vi "Robot Drive Teleop.vi"(9 "Drive Mode":enum16{"Tank Drive", "Arcade Drive"}(ring), 10 "RobotDriveDevRef":T1, 11 "Controller Mode":enum16{"X-Box Controller", "Joysticks"}(ring)) -> (2 "Publish Motors":bool, 3 "Motor Values":dbl[](array[numeric]))   [LabVIEW 2015]
uses:
  <vilib>/Rock Robotics/WPI/RobotDrive/WPI_RobotDriveDevRef.ctl
  <vilib>/Rock Robotics/WPI/MotorControl/WPI_MotorControlDeviceRef.ctl
  <vilib>/Rock Robotics/WPI/MotorControl/WPI_MotorControlType.ctl
  <vilib>/Rock Robotics/SystemInterfaces/DIO/FPGA_DIOPWMChannel.ctl
  <vilib>/Rock Robotics/WPI/PWM/WPI_PWMDeadband.ctl
  <vilib>/Rock Robotics/WPI/CAN/Jaguar/SubVIs/WPI_CANJaguar_ControlMode.ctl
  <vilib>/Rock Robotics/WPI/CAN/TalonSRX/WPI_CANTalonSRX_APIControlMode.ctl
  <vilib>/Rock Robotics/WPI/DriverStation/WPI_DriverStationDerivedRobotMode.ctl
  Robot Global Data.vi
  <vilib>/Rock Robotics/WPI/Utilities/WPI_GetSetVariantRefNum.vi
  <vilib>/Rock Robotics/Network Tables/NT Write Numeric Array.vi
  <vilib>/Rock Robotics/Network Tables/NT Write Boolean Array.vi
panel:
  in  "Buttons":bool[](array[boolean])
  in  "Axes":dbl[](array[numeric])
  in  "POVs":i16[](array[numeric])
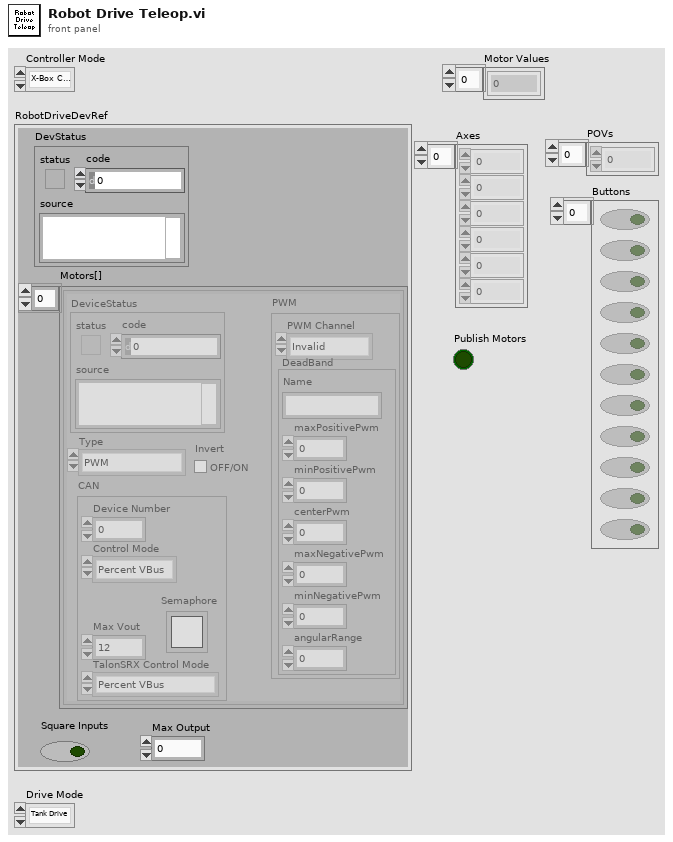
[diagram p1: front panel]
types:
  T1 = typedef "WPI_RobotDriveDevRef.ctl" = cluster{"DevStatus":errorcluster, "Motors[]":T2[], "Square Inputs":bool, "Max Output":dbl}
  T2 = typedef "WPI_MotorControlDeviceRef.ctl" = cluster{"DeviceStatus":errorcluster, "Type":T3, "PWM":cluster{"PWM Channel":T4, "DeadBand":T5}, "CAN":cluster{"Device Number":u8, "Control Mode":T6, "Semaphore":T7, "Max Vout":dbl, "TalonSRX Control Mode":T8}, "Invert":bool}
  T3 = typedef "WPI_MotorControlType.ctl" = enum16{"PWM", "CAN", "CANTalonSRX"}
  T4 = typedef "FPGA_DIOPWMChannel.ctl" = enum8{"PWM 0", "PWM 1", "PWM 2", "PWM 3", "PWM 4", "PWM 5", "PWM 6", "PWM 7", "PWM 8", "PWM 9", "PWM MXP 0", "PWM MXP 1", "PWM MXP 2", "PWM MXP 3", "PWM MXP 4", "PWM MXP 5", "PWM MXP 6", "PWM MXP 7", "PWM MXP 8", "PWM MXP 9", "Invalid"}
  T5 = typedef "WPI_PWMDeadband.ctl" = cluster{"Name":string, "maxPositivePwm":i32, "minPositivePwm":i32, "centerPwm":i32, "maxNegativePwm":i32, "minNegativePwm":i32, "angularRange":u16}
  T6 = typedef "WPI_CANJaguar_ControlMode.ctl" = enum8{"Percent VBus", "Current", "Speed", "Position", "Voltage"}
  T7 = typedef "Semaphore RefNum" = refnum<k1>
  T8 = typedef "WPI_CANTalonSRX_APIControlMode.ctl" = enum8{"Percent VBus", "Speed", "Position", "Slave", "Unchanged / Invalid", "Voltage Compensation", "Current", "Motion Profile"}
  T9 = cluster{"Drive Operation":enum16{"Turn Robot", "Drive Straight for Time"}, "Turn Angle":dbl, "Drive Time":dbl, "Forward Speed":dbl}
  T10 = typedef "WPI_DriverStationDerivedRobotMode.ctl" = enum16{"Init", "Execute", "Stop"}
  T11 = typedef "WPI_JoystickDevRef.ctl" = cluster{"Device":T12}
  T12 = typedef "WPI_JoystickDeviceEnum.ctl" = enum16{"USB 0", "USB 1", "USB 2", "USB 3", "USB 4", "USB 5"}
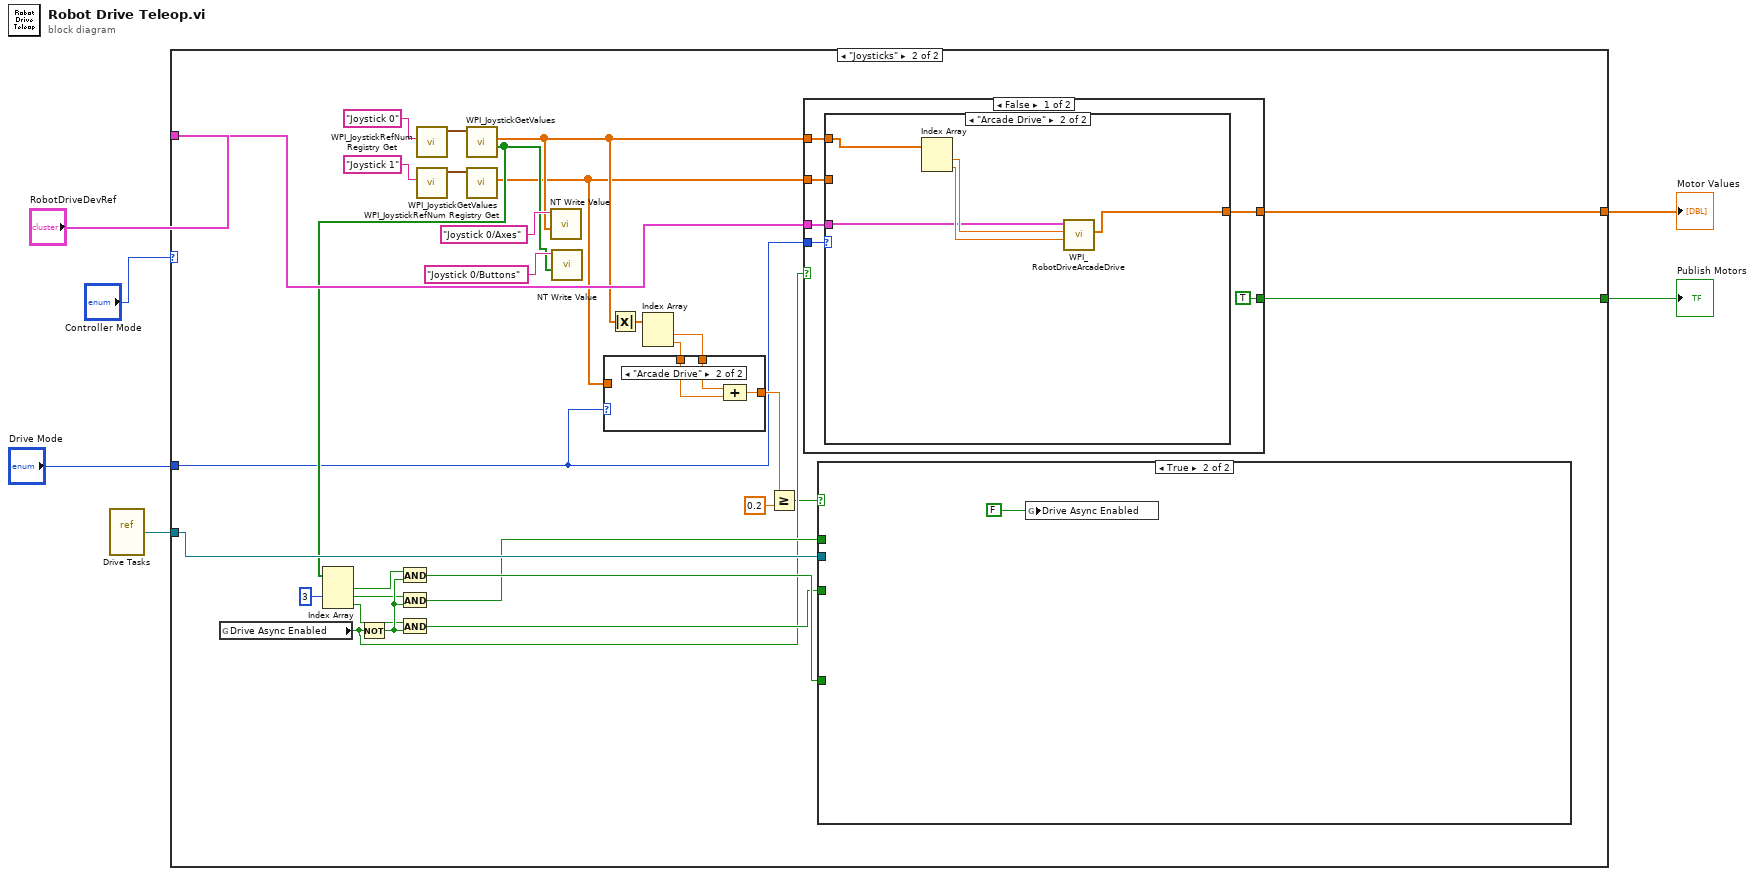
[diagram p0: block diagram]
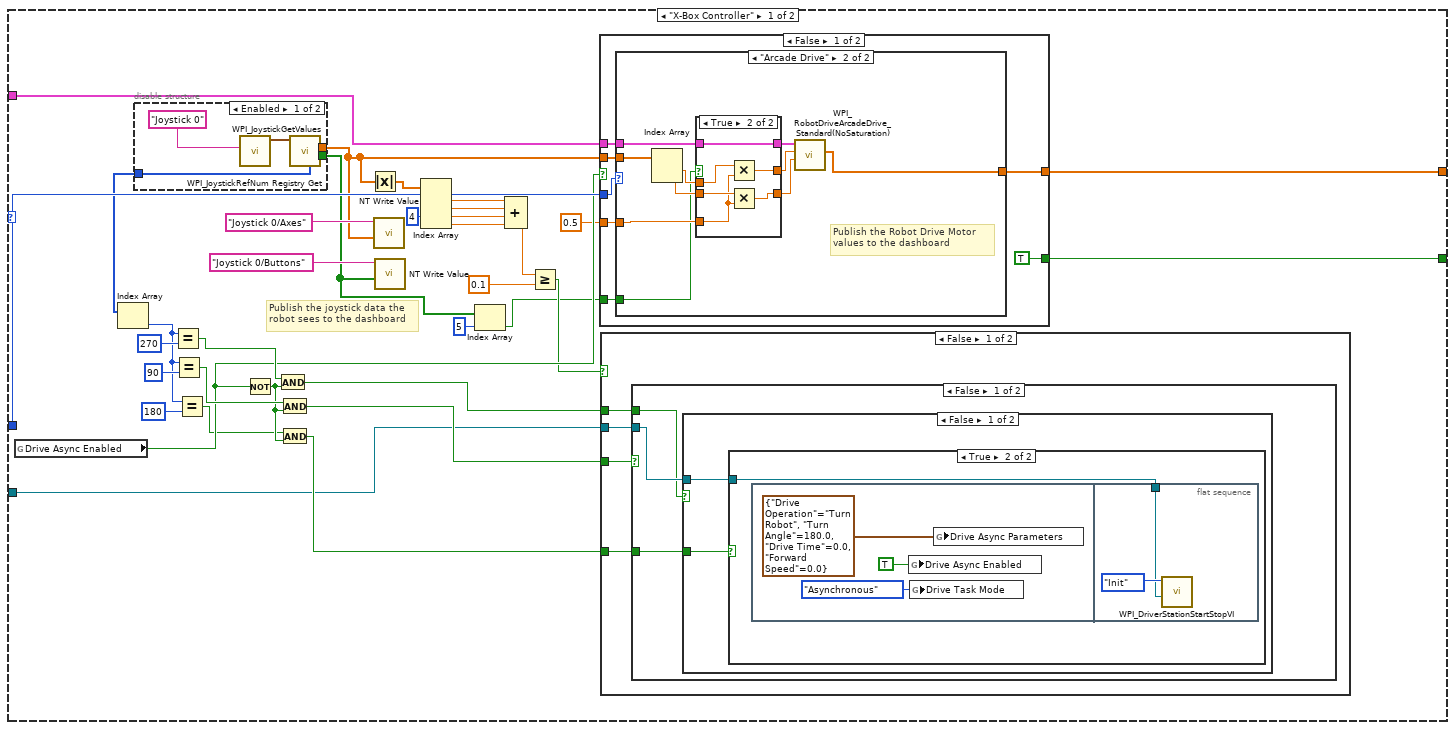
[diagram p2: hidden frame]
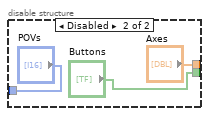
[diagram p3: hidden frame]
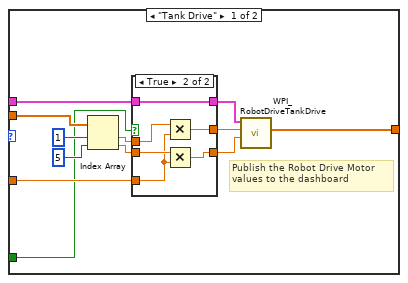
[diagram p4: hidden frame]
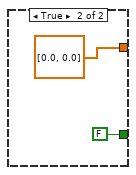
[diagram p7: hidden frame]
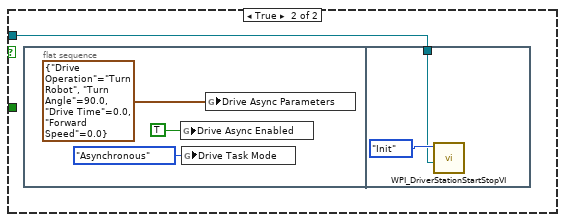
[diagram p9: hidden frame]
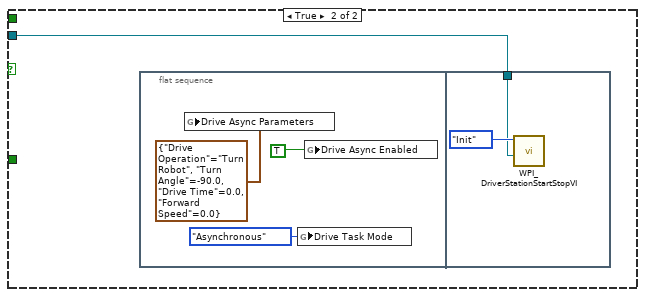
[diagram p10: hidden frame]
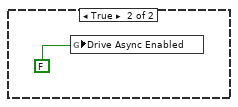
[diagram p11: hidden frame]
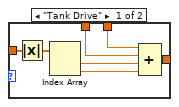
[diagram p12: hidden frame]
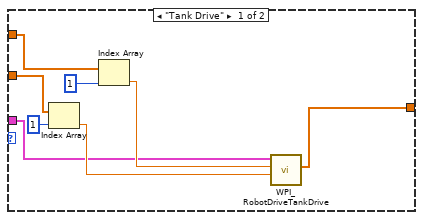
[diagram p13: hidden frame]
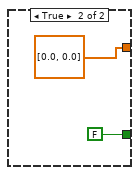
[diagram p14: hidden frame]
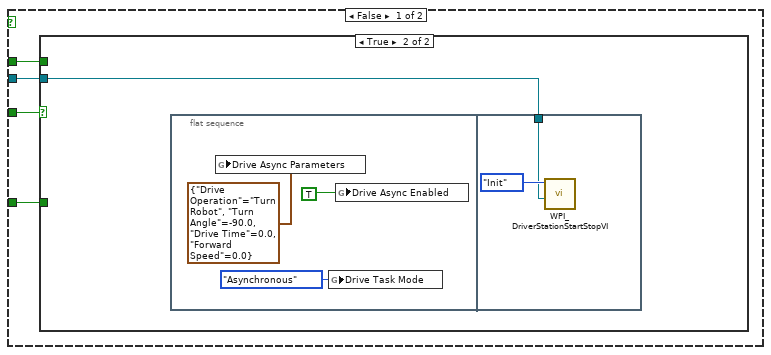
[diagram p15: hidden frame]
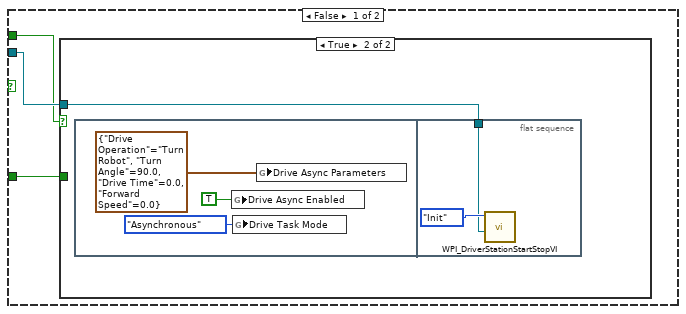
[diagram p16: hidden frame]
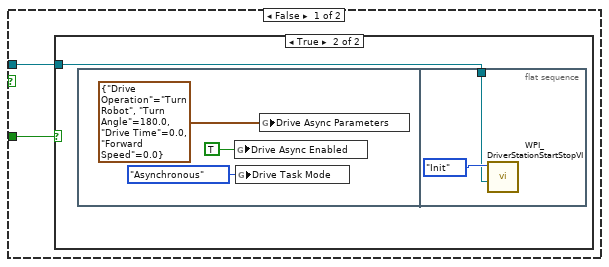
[diagram p17: hidden frame]
diagram:
  n1 = vi-ref "Drive Tasks.vi"() -> (w1:refnum<vi>)
  n2 = case shown="\"Joysticks\"" "Controller Mode" {
    tunnel: "RobotDriveDevRef" -> [w38 w148]
    tunnel: "Drive Mode" -> [w37 w126]
    tunnel: [w36 w147] -> w6
    tunnel: [w17 w135] -> w2
    tunnel: w1 -> [w11 w146]
    frame "X-Box Controller" {
      # "Publish the joystick data the\nrobot sees to the dashboard"
      n3 = global read "Robot Global Data.vi" "Drive Async Enabled"() -> (w20:bool)
      n4 = disable-structure shown="Enabled" {
        disable-tunnel: [w43 "Buttons"] -> w9
        disable-tunnel: [w42 "Axes"] -> w29
        disable-tunnel: [w41 "POVs"] -> w26
        frame Enabled {
          n5 = call <vilib>:"WPI_JoystickRefNum Registry Get.vi"("refnum name"="Joystick 0") -> ("JoystickDevRef"=w44:T11)  [unwired: 1 in, 9 out]
          n6 = call <vilib>:"WPI_JoystickGetValues.vi"("JoystickDevRef"=w44) -> ("Buttons"=w43:bool[], "Axes"=w42:dbl[], "POVs"=w41:i16[])  [unwired: 6 in, 2 out]
        }
        frame Disabled {
        }
      }
      n7 = Index Array(array=w26) -> (element=w15:i16)  [unwired: 1 in]
      n8 = Equal?(x=w15, y=i16 270) -> (x = y?=w24:bool)
      n9 = Equal?(x=w15, y=i16 90) -> (x = y?=w22:bool)
      n10 = Equal?(x=w15, y=i16 180) -> (x = y?=w13:bool)
      n11 = Not(x=w20) -> (.not. x?=w14:bool)
      n12 = And(x=w24, y=w14) -> (x .and. y?=w19:bool)
      n13 = And(x=w22, y=w14) -> (x .and. y?=w21:bool)
      n14 = And(x=w13, y=w14) -> (x .and. y?=w12:bool)
      n15 = Absolute Value(x=w29) -> (abs(x)=w30:dbl[])
      n16 = call-poly <vilib>:"NT Write Value.vi"("Numeric Array"=w29, "Name"="Joystick 0/Axes") -> ()  [unwired: 9 in, 1 out]
      n17 = call-poly <vilib>:"NT Write Value.vi"("Boolean Array"=w9, "Name"="Joystick 0/Buttons") -> ()  [unwired: 9 in, 1 out]
      n18 = Index Array(array=w30, index #3=4 ("index")) -> (element #1=w34:dbl, element #2=w33:dbl, element #3=w32:dbl, element #4=w31:dbl)  [unwired: 3 in]
      n19 = Index Array(array=w9, index=5) -> (element=w7:bool)
      n20 = Compound Arithmetic op=ADD(w34, w33, w32, w31) -> (w28:dbl)
      n21 = Greater Or Equal?(x=w28, y=0.1) -> (x >= y?=w18:bool)
      n22 = case shown="False" w20 {
        tunnel: w38 -> [w55 _]
        tunnel: w37 -> [w54 _]
        tunnel: [w53 dbl[] [0.0, 0.0] ("Motor Values")] -> w36
        tunnel: w29 -> [w52 _]
        tunnel: [TRUE FALSE] -> w17
        tunnel: 0.5 -> [w50 _]
        tunnel: w7 -> [w49 _]
        frame False {
          n23 = case shown="\"Arcade Drive\"" w54 {
            tunnel: w55 -> [w57 w78]
            tunnel: w52 -> [w65 w86]
            tunnel: [w64 w85] -> w53
            tunnel: w50 -> [w59 w83]
            tunnel: w49 -> [w56 w77]
            frame "Tank Drive" {
              # "Publish the Robot Drive Motor\nvalues to the dashboard"
              n24 = Index Array(array=w65, index #1=1 ("index"), index #2=5 ("index")) -> (element #1=w62:dbl, element #2=w60:dbl)
              n25 = case shown="True" w56 {
                tunnel: [w70 w76] -> w63
                tunnel: w62 -> [w70 w75]
                tunnel: [w69 w73] -> w61
                tunnel: w60 -> [w69 w74]
                tunnel: w59 -> [_ w72]
                tunnel: [w68 w71] -> w58
                tunnel: w57 -> [w68 w71]
                frame False {
                }
                frame True {
                  n26 = Multiply(x=w75, y=w72) -> (x*y=w76:dbl)
                  n27 = Multiply(x=w74, y=w72) -> (x*y=w73:dbl)
                }
              }
              n28 = call <vilib>:"WPI_RobotDriveTankDrive.vi"("Right axis value"=w61, "Left axis value"=w63, "RobotDriveDevRef"=w58) -> ("Motor Values"=w64:dbl[])  [unwired: 6 in, 2 out]
            }
            frame "Arcade Drive" {
              # "Publish the Robot Drive Motor\nvalues to the dashboard"
              n29 = Index Array(array=w86) -> (element #1=w84:dbl, element #2=w80:dbl)  [unwired: 2 in]
              n30 = case shown="True" w77 {
                tunnel: [w89 w95] -> w82
                tunnel: w84 -> [w89 w94]
                tunnel: [w88 w92] -> w81
                tunnel: w80 -> [w88 w93]
                tunnel: w83 -> [_ w91]
                tunnel: [w87 w90] -> w79
                tunnel: w78 -> [w87 w90]
                frame False {
                }
                frame True {
                  n31 = Multiply(x=w94, y=w91) -> (x*y=w95:dbl)
                  n32 = Multiply(x=w93, y=w91) -> (x*y=w92:dbl)
                }
              }
              n33 = call <vilib>:"WPI_RobotDriveArcadeDrive_Standard(NoSaturation).vi"("Y axis value"=w81, "X axis value"=w82, "RobotDriveDevRef"=w79) -> ("Motor Values"=w85:dbl[])  [unwired: 1 in, 7 out]
            }
          }
        }
        frame True {
        }
      }
      n34 = case shown="False" w18 {
        tunnel: w11 -> [w101 _]
        tunnel: w21 -> [w100 _]
        tunnel: w19 -> [w99 _]
        tunnel: w12 -> [w98 _]
        frame False {
          n35 = case shown="False" w100 {
            tunnel: w101 -> [w104 w119]
            tunnel: w99 -> [w103 _]
            tunnel: w98 -> [w102 _]
            frame False {
              n36 = case shown="False" w103 {
                tunnel: w104 -> [w105 w113]
                tunnel: w102 -> [w106 _]
                frame False {
                  n37 = case shown="True" w106 {
                    tunnel: w105 -> [_ w107]
                    frame False {
                    }
                    frame True {
                      n38 = flat-sequence {
                        tunnel: w107 -> [w111]
                        frame #0 {
                          n39 = global write "Robot Global Data.vi" "Drive Async Enabled"(TRUE ("Drive Async")) -> ()
                          n40 = global write "Robot Global Data.vi" "Drive Task Mode"(enum16{"Synchronous", "Asynchronous"}."Asynchronous" ("Drive Task Mode")) -> ()
                          n41 = global write "Robot Global Data.vi" "Drive Async Parameters"(T9 {"Drive Operation"=enum."Turn Robot", "Turn Angle"=180.0, "Drive Time"=0.0, "Forward Speed"=0.0} ("Drive Async Parameters")) -> ()
                        }
                        frame #1 {
                          n42 = call <vilib>:"WPI_DriverStationStartStopVI.vi"("VI in"=w111, "Call Context"=WPI_DriverStationDerivedRobotMode."Init") -> ()  [unwired: 10 in]
                        }
                      }
                    }
                  }
                }
                frame True {
                  n43 = flat-sequence {
                    tunnel: w113 -> [w117]
                    frame #0 {
                      n44 = global write "Robot Global Data.vi" "Drive Async Enabled"(TRUE ("Drive Async")) -> ()
                      n45 = global write "Robot Global Data.vi" "Drive Task Mode"(enum16{"Synchronous", "Asynchronous"}."Asynchronous" ("Drive Task Mode")) -> ()
                      n46 = global write "Robot Global Data.vi" "Drive Async Parameters"(T9 {"Drive Operation"=enum."Turn Robot", "Turn Angle"=90.0, "Drive Time"=0.0, "Forward Speed"=0.0} ("Drive Async Parameters")) -> ()
                    }
                    frame #1 {
                      n47 = call <vilib>:"WPI_DriverStationStartStopVI.vi"("VI in"=w117, "Call Context"=WPI_DriverStationDerivedRobotMode."Init") -> ()  [unwired: 10 in]
                    }
                  }
                }
              }
            }
            frame True {
              n48 = flat-sequence {
                tunnel: w119 -> [w123]
                frame #0 {
                  n49 = global write "Robot Global Data.vi" "Drive Async Parameters"(T9 {"Drive Operation"=enum."Turn Robot", "Turn Angle"=-90.0, "Drive Time"=0.0, "Forward Speed"=0.0} ("Drive Async Parameters")) -> ()
                  n50 = global write "Robot Global Data.vi" "Drive Task Mode"(enum16{"Synchronous", "Asynchronous"}."Asynchronous" ("Drive Task Mode")) -> ()
                  n51 = global write "Robot Global Data.vi" "Drive Async Enabled"(TRUE ("Drive Async")) -> ()
                }
                frame #1 {
                  n52 = call <vilib>:"WPI_DriverStationStartStopVI.vi"("VI in"=w123, "Call Context"=WPI_DriverStationDerivedRobotMode."Init") -> ()  [unwired: 10 in]
                }
              }
            }
          }
        }
        frame True {
          n53 = global write "Robot Global Data.vi" "Drive Async Enabled"(FALSE ("Drive Async")) -> ()
        }
      }
    }
    frame "Joysticks" {
      n54 = global read "Robot Global Data.vi" "Drive Async Enabled"() -> (w136:bool)
      n55 = Not(x=w136) -> (.not. x?=w145:bool)
      n56 = call <vilib>:"WPI_JoystickRefNum Registry Get.vi"("refnum name"="Joystick 0") -> ("JoystickDevRef"=w153:T11)  [unwired: 1 in, 9 out]
      n57 = call <vilib>:"WPI_JoystickRefNum Registry Get.vi"("refnum name"="Joystick 1") -> ("JoystickDevRef"=w149:T11)  [unwired: 1 in, 9 out]
      n58 = call <vilib>:"WPI_JoystickGetValues.vi"("JoystickDevRef"=w153) -> ("Buttons"=w144:bool[], "Axes"=w128:dbl[])  [unwired: 6 in, 3 out]
      n59 = Index Array(array=w144, index #2=3 ("index")) -> (element #1=w142:bool, element #2=w141:bool, element #3=w140:bool)  [unwired: 2 in]
      n60 = And(x=w142, y=w145) -> (x .and. y?=w139:bool)
      n61 = And(x=w141, y=w145) -> (x .and. y?=w138:bool)
      n62 = And(x=w140, y=w145) -> (x .and. y?=w137:bool)
      n63 = call <vilib>:"WPI_JoystickGetValues.vi"("JoystickDevRef"=w149) -> ("Axes"=w127:dbl[])  [unwired: 6 in, 4 out]
      n64 = call-poly <vilib>:"NT Write Value.vi"("Numeric Array"=w128, "Name"="Joystick 0/Axes") -> ()  [unwired: 9 in, 1 out]
      n65 = call-poly <vilib>:"NT Write Value.vi"("Boolean Array"=w144, "Name"="Joystick 0/Buttons") -> ()  [unwired: 9 in, 1 out]
      n66 = Absolute Value(x=w128) -> (abs(x)=w132:dbl[])
      n67 = Index Array(array=w132) -> (element #1=w134:dbl, element #2=w133:dbl)  [unwired: 2 in]
      n68 = case shown="\"Arcade Drive\"" w126 {
        tunnel: w134 -> [w161 w164]
        tunnel: w133 -> [w160 w163]
        tunnel: [w156 w162] -> w130
        tunnel: w127 -> [w155 _]
        frame "Tank Drive" {
          n69 = Absolute Value(x=w155) -> (abs(x)=w157:dbl[])
          n70 = Index Array(array=w157) -> (element #1=w159:dbl, element #2=w158:dbl)  [unwired: 2 in]
          n71 = Compound Arithmetic op=ADD(w161, w160, w159, w158) -> (w156:dbl)
        }
        frame "Arcade Drive" {
          n72 = Compound Arithmetic op=ADD(w164, w163) -> (w162:dbl)
        }
      }
      n73 = Greater Or Equal?(x=w130, y=0.2) -> (x >= y?=w129:bool)
      n74 = case shown="False" w136 {
        tunnel: w126 -> [w170 _]
        tunnel: w128 -> [w169 _]
        tunnel: w127 -> [w168 _]
        tunnel: w148 -> [w167 _]
        tunnel: [w166 dbl[] [0.0, 0.0] ("Motor Values")] -> w147
        tunnel: [TRUE FALSE] -> w135
        frame False {
          n75 = case shown="\"Arcade Drive\"" w170 {
            tunnel: w169 -> [w173 w180]
            tunnel: w168 -> [w172 _]
            tunnel: w167 -> [w174 w181]
            tunnel: [w171 w179] -> w166
            frame "Tank Drive" {
              n76 = Index Array(array=w172, index=1) -> (element=w175:dbl)
              n77 = Index Array(array=w173, index=1) -> (element=w176:dbl)
              n78 = call <vilib>:"WPI_RobotDriveTankDrive.vi"("Right axis value"=w175, "Left axis value"=w176, "RobotDriveDevRef"=w174) -> ("Motor Values"=w171:dbl[])  [unwired: 6 in, 2 out]
            }
            frame "Arcade Drive" {
              n79 = Index Array(array=w180) -> (element #1=w183:dbl, element #2=w182:dbl)  [unwired: 2 in]
              n80 = call-poly <vilib>:"WPI_RobotDriveArcadeDrive.vi"("Y axis value"=w182, "X axis value"=w183, "RobotDriveDevRef"=w181) -> ("Motor Values"=w179:dbl[])  [unwired: 6 in, 2 out]
            }
          }
        }
        frame True {
        }
      }
      n81 = case shown="True" w129 {
        tunnel: w146 -> [w189 _]
        tunnel: w137 -> [w188 _]
        tunnel: w138 -> [w187 _]
        tunnel: w139 -> [w186 _]
        frame False {
          n82 = case shown="True" w188 {
            tunnel: w189 -> [w192 w207]
            tunnel: w187 -> [w191 _]
            tunnel: w186 -> [w190 _]
            frame False {
              n83 = case shown="True" w191 {
                tunnel: w192 -> [w193 w201]
                tunnel: w190 -> [w194 _]
                frame False {
                  n84 = case shown="True" w194 {
                    tunnel: w193 -> [_ w195]
                    frame False {
                    }
                    frame True {
                      n85 = flat-sequence {
                        tunnel: w195 -> [w199]
                        frame #0 {
                          n86 = global write "Robot Global Data.vi" "Drive Async Enabled"(TRUE ("Drive Async")) -> ()
                          n87 = global write "Robot Global Data.vi" "Drive Task Mode"(enum16{"Synchronous", "Asynchronous"}."Asynchronous" ("Drive Task Mode")) -> ()
                          n88 = global write "Robot Global Data.vi" "Drive Async Parameters"(T9 {"Drive Operation"=enum."Turn Robot", "Turn Angle"=180.0, "Drive Time"=0.0, "Forward Speed"=0.0} ("Drive Async Parameters")) -> ()
                        }
                        frame #1 {
                          n89 = call <vilib>:"WPI_DriverStationStartStopVI.vi"("VI in"=w199, "Call Context"=WPI_DriverStationDerivedRobotMode."Init") -> ()  [unwired: 10 in]
                        }
                      }
                    }
                  }
                }
                frame True {
                  n90 = flat-sequence {
                    tunnel: w201 -> [w205]
                    frame #0 {
                      n91 = global write "Robot Global Data.vi" "Drive Async Enabled"(TRUE ("Drive Async")) -> ()
                      n92 = global write "Robot Global Data.vi" "Drive Task Mode"(enum16{"Synchronous", "Asynchronous"}."Asynchronous" ("Drive Task Mode")) -> ()
                      n93 = global write "Robot Global Data.vi" "Drive Async Parameters"(T9 {"Drive Operation"=enum."Turn Robot", "Turn Angle"=90.0, "Drive Time"=0.0, "Forward Speed"=0.0} ("Drive Async Parameters")) -> ()
                    }
                    frame #1 {
                      n94 = call <vilib>:"WPI_DriverStationStartStopVI.vi"("VI in"=w205, "Call Context"=WPI_DriverStationDerivedRobotMode."Init") -> ()  [unwired: 10 in]
                    }
                  }
                }
              }
            }
            frame True {
              n95 = flat-sequence {
                tunnel: w207 -> [w211]
                frame #0 {
                  n96 = global write "Robot Global Data.vi" "Drive Async Parameters"(T9 {"Drive Operation"=enum."Turn Robot", "Turn Angle"=-90.0, "Drive Time"=0.0, "Forward Speed"=0.0} ("Drive Async Parameters")) -> ()
                  n97 = global write "Robot Global Data.vi" "Drive Task Mode"(enum16{"Synchronous", "Asynchronous"}."Asynchronous" ("Drive Task Mode")) -> ()
                  n98 = global write "Robot Global Data.vi" "Drive Async Enabled"(TRUE ("Drive Async")) -> ()
                }
                frame #1 {
                  n99 = call <vilib>:"WPI_DriverStationStartStopVI.vi"("VI in"=w211, "Call Context"=WPI_DriverStationDerivedRobotMode."Init") -> ()  [unwired: 10 in]
                }
              }
            }
          }
        }
        frame True {
          n100 = global write "Robot Global Data.vi" "Drive Async Enabled"(FALSE ("Drive Async")) -> ()
        }
      }
    }
  }
  "Motor Values" <- w6
  "Publish Motors" <- w2
